vi "Set 仪器电源.vi"(10 "仪器电源":refnum<vi>, 11 "DAM0200-Relay in":refnum<class "DAM0200-Relay.lvclass">) -> (3 "DAM0200-Relay out":refnum<class "DAM0200-Relay.lvclass">)   [LabVIEW 2016, in "DAM0200-Relay.lvlib" / "DAM0200-Relay.lvclass"]
uses:
  DAM0200-Relay.lvclass
  DAM0200-Relay.lvclass/DAM0200-Relay.ctl
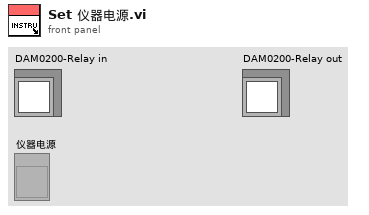
[diagram p1: front panel]
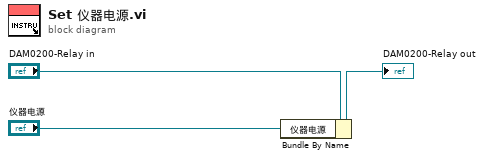
[diagram p0: block diagram]
diagram:
  n1 = Bundle By Name(cluster="DAM0200-Relay in", "仪器电源"="仪器电源") -> (→"DAM0200-Relay out":refnum<class "DAM0200-Relay.lvclass">)
